vi "Actor Core.vi"(8 "error in":errorcluster, 11 "Normal Car Wash Status View In":refnum<class "Normal Car Wash Status View.lvclass">) -> (0 "error out":errorcluster, 3 "Actor out":refnum<class "Actor.lvclass">)   [LabVIEW 2019, in "Normal Car Wash Status View.lvclass"]
doc: "(<B>Filename</B>: Actor Framework.lvlib:Actor.lvclass:Actor Core.vi)\n\nReceives messages to the actor, reacts to them, and initiates any error handling that may shut the actor down.\n\nDescendant classes may override this VI to append parallel tasks for the actor to complete while it handles messages. Overrides use the Call Parent Method node.\n\n<License>\nCopyright © 2017 Composed Systems, LLC | All rights reserved\nwww.composed.io\n\nAuthor: Ethan Stern <ethan.stern@composed.io>\n\nThis software is provided \"AS IS\" WITHOUT WARRANTIES, either express or implied, AND IS FOR EDUCATIONAL PURPOSES ONLY.\n</License>"
uses:
  <vilib>/gpm_packages/@cs/Car-wash/Source/Normal Car Wash Status View/Normal Car Wash Status View/Normal Car Wash Status View.lvclass
  <vilib>/gpm_packages/@cs/Car-wash/Source/Car Wash Status View Definition/Car Wash Status View Definition/Car Wash Status View Definition.lvclass
  C:/Program Files/National Instruments/LabVIEW 2019/vi.lib/gpm_packages/@cs/composed-car-wash/Source/Car Wash Status View Definition/Car Wash Status View Definition/Car Wash Status View Definition.lvclass
  C:/Program Files/National Instruments/LabVIEW 2019/vi.lib/gpm_packages/@cs/mva-viewable/Source/IViewable/IViewable/IViewable.lvclass
  C:/Program Files/National Instruments/LabVIEW 2019/vi.lib/gpm_packages/@cs/mva-viewable/Source/ActorEvents/IEventAggregator/IEventAggregator.lvclass
  C:/Program Files/National Instruments/LabVIEW 2019/vi.lib/gpm_packages/@cs/mva-core/Source/IObserver/IObserver/IObserver.lvclass
  C:/Program Files/National Instruments/LabVIEW 2019/vi.lib/ActorFramework/Actor/Actor.lvclass
  <vilib>/ActorFramework/Actor/Actor.lvclass
panel:
  out "Wash Entry State":bool caption="Wash Entry"
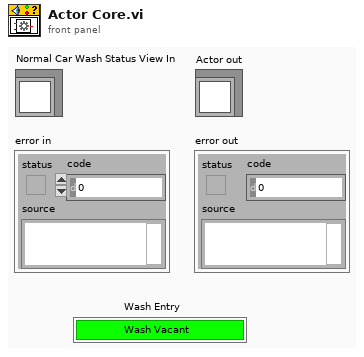
[diagram p1: front panel]
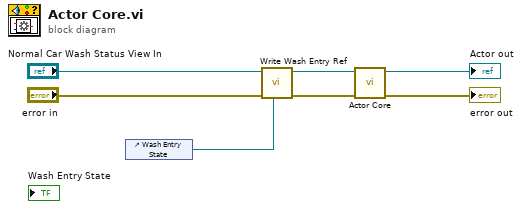
[diagram p0: block diagram]
diagram:
  n1 = control-ref of="Wash Entry State"() -> (w1:refnum<vi>)
  n2 = call <vilib>:"Write Wash Entry Ref.vi"("Wash Entry Ref"=w1, "Car Wash Status View Definition in"="Normal Car Wash Status View In") -> ("Car Wash Status View Definition out"=w2:refnum<class "Normal Car Wash Status View.lvclass">)  [unwired: 9 in]
  n3 = call-parent "Actor Core.vi"("error in"="error in", "Car Wash Status View Definition In"=w2) -> ("error out"=→"error out":errorcluster, "Actor out"=→"Actor out":refnum<class "Actor.lvclass">)  [unwired: 8 in]
